vi "V to Deg.vi"(1 "Voltaje de entrada (0-5V)":dbl, 3 "error in (no error)":errorcluster) -> (7 "Angulo [-135, 135]":dbl(knob) scale=-135.0..135.0, 10 "error out":errorcluster)   [LabVIEW 2018]
uses:
  <vilib>/gmath/NI_Gmath.lvlib
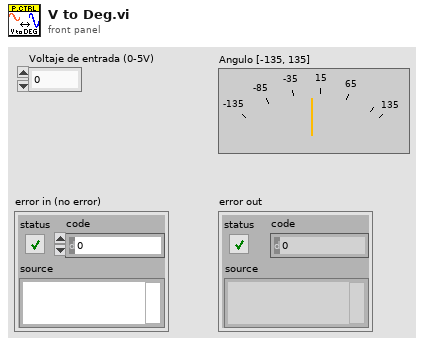
[diagram p1: front panel]
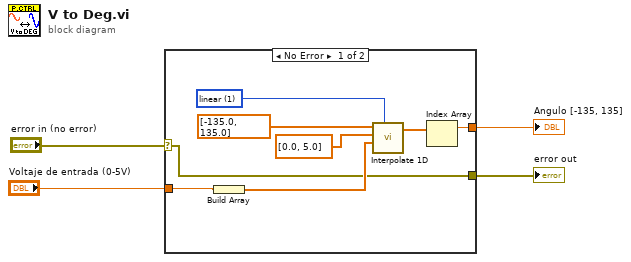
[diagram p0: block diagram]
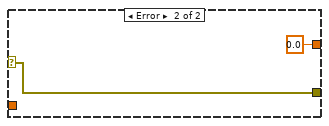
[diagram p2: hidden frame]
diagram:
  n1 = case shown="No Error" "error in (no error)" {
    selector: "error in (no error)" -> [w5 w14]
    tunnel: [w12 0.0 ("Numeric")] -> w4
    tunnel: "Voltaje de entrada (0-5V)" -> [w10 _]
    tunnel: [w5 w14] -> w1
    frame No Error {
      w6 = 1 items=["nearest", "linear", "spline", "cubic Hermite", "Lagrange"] ("method")
      n2 = Build Array(w10) -> (w7:dbl[])
      n3 = call <vilib>:"Interpolate 1D.vi"("method"=w6, "xi"=w7, "X"=dbl[] [0.0, 5.0], "Y"=dbl[] [-135.0, 135.0]) -> ("yi"=w11:dbl[])  [unwired: 5 in, 2 out]
      n4 = Index Array(array=w11) -> (element=w12:dbl)  [unwired: 1 in]
    }
    frame Error {
    }
  }
  "Angulo [-135, 135]" <- w4
  "error out" <- w1
